vi "Increment String.vi"(9 "Numeric":u32, 10 "Input String":string, 11 "String Increment Algorithm":refnum<class "StringIncrementAlgorithm.lvclass">) -> (2 "Incremented String":string)   [LabVIEW 2014, in "StringIncrementAlgorithm.lvclass"]
uses:
  StringIncrementAlgorithm.lvclass
  StringIncrementAlgorithm.lvclass/StringIncrementAlgorithm.ctl
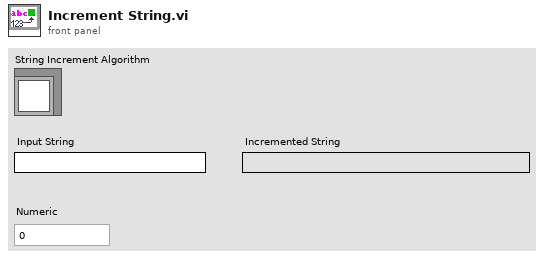
[diagram p1: front panel]
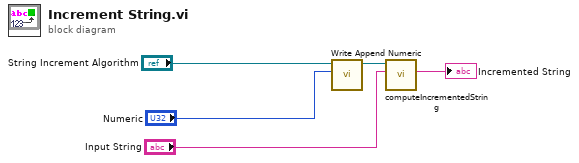
[diagram p0: block diagram]
diagram:
  n1 = call "Write Append Numeric.vi"("Append Numeric"="Numeric", "StringIncrementAlgorithm in"="String Increment Algorithm") -> ("StringIncrementAlgorithm out"=w3:refnum<class "StringIncrementAlgorithm.lvclass">)  [unwired: 9 in]
  n2 = call-dynamic "computeIncrementedString.vi"("Input String"="Input String", "StringIncrementAlgorithm in"=w3) -> ("Incremented String"=→"Incremented String":string)  [unwired: 8 in, 1 out]
